vi "UV-VIS GetNumberVSSpeedsSD.vi"(4 "error in (no error)":errorcluster, 7 "Control in":refnum<class "CCD_camera.lvclass">) -> (0 "error out":errorcluster, 1 "DLL error code":u32, 2 "number":i32, 3 "Control out":refnum<class "CCD_camera.lvclass">)   [LabVIEW 2020, in "CCD_camera.lvclass"]
doc: "As your AndorMCD[tm] system may be capable of operating at more than one vertical shift speed this function will return the actual number of speeds available.\n\n<B>Parameter:</B>\nnumber - number of allowed vertical speeds\n\n<B>Error codes:</B>\nDRV_SUCCESS - Number of speeds returned.\nDRV_NOT_INITIALIZED - System not initialized.\nDRV_ACQUIRING - Acquisition in progress.\n\n<B>NOTES:</B>\n<B>Can also be used during ‘Run Till Abort’ Mode.</B>"
uses:
  CCD_camera.lvclass
  C:/dev/TRANCON/Classes/Detector/Detector.lvclass
  Detector.lvclass/Detector.ctl
  Detector.lvclass
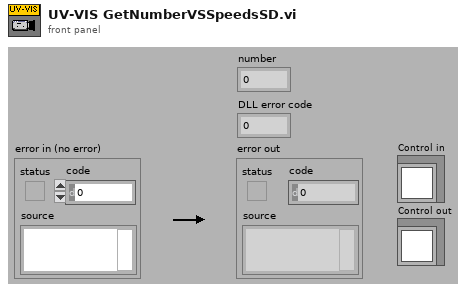
[diagram p1: front panel]
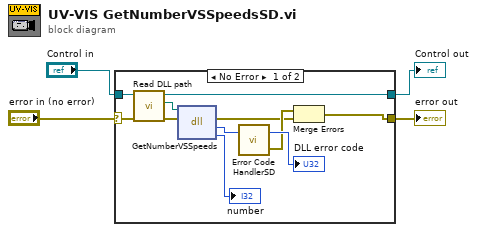
[diagram p0: block diagram]
diagram:
  n1 = case shown="No Error" "error in (no error)" {
    selector: "error in (no error)" -> [w9 w17]
    tunnel: [w6 w17] -> w3
    tunnel: [w5 w16] -> w2
    tunnel: "Control in" -> [w10 w16]
    frame No Error {
      n2 = call "Read DLL path.vi"("error in (no error)"=w9, "Detector in"=w10) -> ("error out"=w11:errorcluster, "DLL path"=w8:path, "Detector out"=w5:refnum<class "CCD_camera.lvclass">)  [unwired: 7 in]
      n3 = dll-call lib="S:/TRANCON/DLL/Atmcd32d.dll" fn="GetNumberVSSpeeds"(path in=w8, error in=w11) -> (error out=w7:errorcluster, "return type"=w15:u32, "number"=→"number":i32)  [unwired: 2 in, 1 out]
      n4 = call "Error Code HandlerSD.vi"("DLL error code"=w15) -> ("error out"=w12:errorcluster, "dup DLL error code"=→"DLL error code":u32)  [unwired: 1 in]
      n5 = Merge Errors(w12, w7) -> (w6:errorcluster)
    }
    frame Error {
    }
  }
  "error out" <- w3
  "Control out" <- w2
